vi "arraysX to String Array.vi"(0 "format string":string, 2 "Array 6":sgl[](array[numeric])) -> (14 "Array":string[](array[string]))   [LabVIEW 2021]
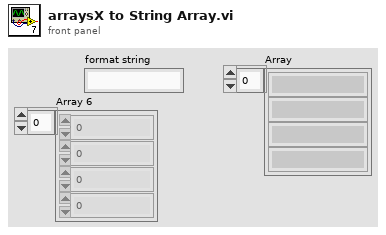
[diagram p1: front panel]
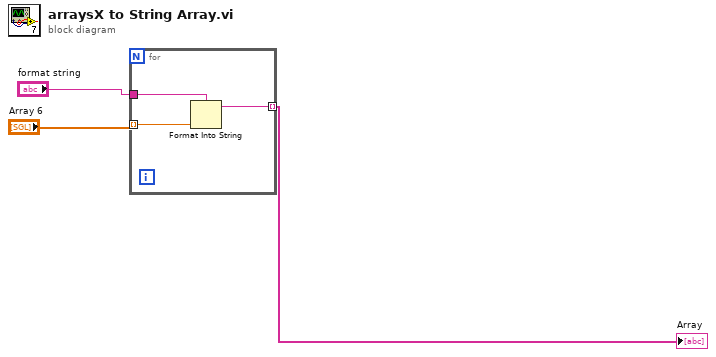
[diagram p0: block diagram]
diagram:
  n1 = for {
    tunnel: "Array 6" -> [w4] mode=indexing
    tunnel: [w6] -> w2 mode=indexing
    tunnel: "format string" -> [w5]
    n2 = Format Into String(format string=w5, w4) -> (resulting string=w6:string)  [unwired: 2 in, 1 out]
  }
  "Array" <- w2
